vi "Duplicate_DO_WF.vi"(8 "error in":errorcluster) -> (0 "error out":errorcluster, 3 "Digital waveform 3":digitalwaveform[](graph))   [LabVIEW 2025]
uses:
  <vilib>/Waveform/DWDTOps.llb/DWDT Digital Size.vi
  <vilib>/Waveform/DWDTOps.llb/DWDT Append Digital Samples.vi
panel:
  out "Samples":u32
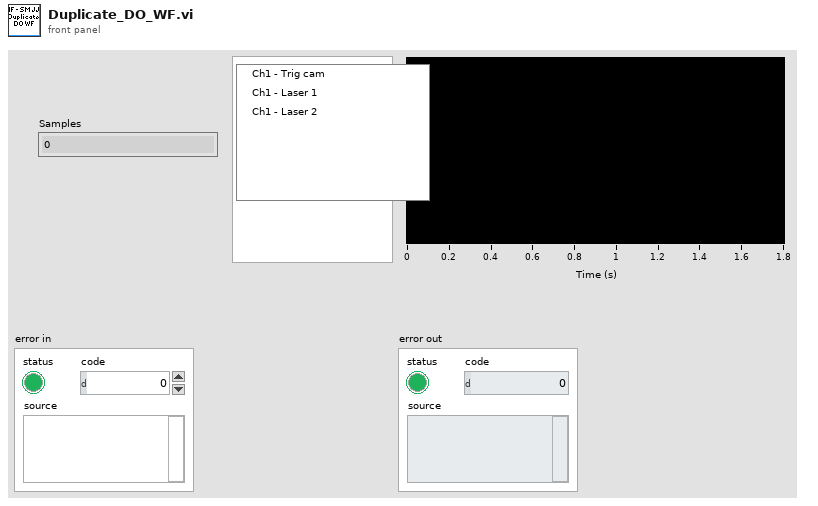
[diagram p1: front panel]
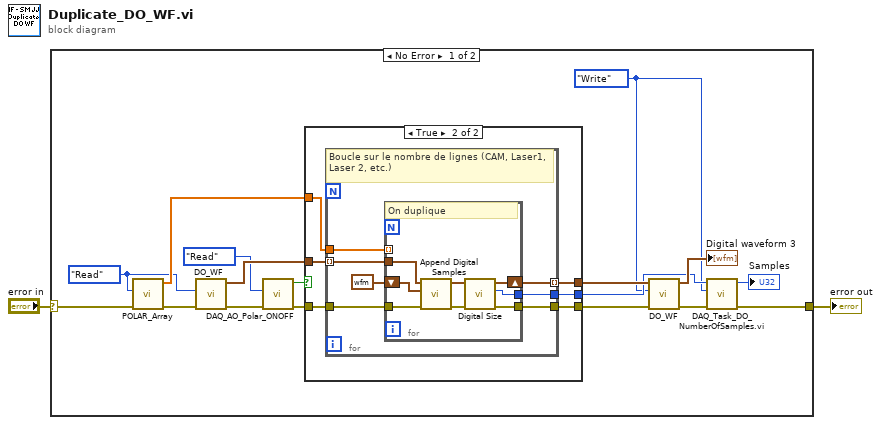
[diagram p0: block diagram]
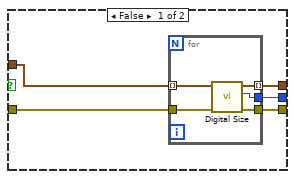
[diagram p2: hidden frame]
diagram:
  n1 = case shown="No Error" "error in" {
    selector: "error in" -> [w16 w51]
    tunnel: [w9 w51] -> w1
    frame No Error {
      w8 = enum16{"Init", "Write", "Read"}."Write" ("Action")
      w7 = enum16{"Init", "Write", "Read"}."Read" ("Action")
      n2 = call "POLAR_Array.vi"("error in"=w16, "Action"=w7) -> ("error out"=w15:errorcluster, "Pockels_Array"=w14:dbl[])  [unwired: 8 in]
      n3 = call "DO_WF.vi"("error in"=w15, "Action"=w7) -> ("error out"=w6:errorcluster, "Digital WF"=w19:digitalwaveform[])  [unwired: 8 in]
      n4 = call "DAQ_AO_Polar_ONOFF.vi"("error in"=w6, "Action"=enum16{"Init", "Write", "Read"}."Read") -> ("error out"=w5:errorcluster, "ON / OFF"=w3:bool)  [unwired: 8 in]
      n5 = case shown="True" w3 {
        tunnel: w19 -> [w24 w35]
        tunnel: [w22 w34] -> w18
        tunnel: w14 -> [_ w33]
        tunnel: [w20 w32] -> w13
        tunnel: [w23 w31] -> w12
        tunnel: w5 -> [w21 w30]
        frame False {
          n6 = for {
            tunnel: w24 -> [w29] mode=indexing
            tunnel: [w28] -> w23
            tunnel: [w27] -> w22
            tunnel: w21 -> [w26]
            tunnel: [w25] -> w20 mode=indexing
            n7 = call-poly <vilib>:"Digital Size.vi"("error in (no error)"=w26, "digital waveform in"=w29) -> ("error out"=w27:errorcluster, "number of samples"=w28:i32, "digital waveform out"=w25:digitalwaveform)  [unwired: 6 in, 1 out]
          }
        }
        frame True {
          n8 = for {
            tunnel: w35 -> [w42] mode=indexing
            tunnel: [w37] -> w32 mode=indexing
            tunnel: w33 -> [w40]
            tunnel: [w36] -> w31
            tunnel: w30 -> [w39]
            tunnel: [w38] -> w34
            # "Boucle sur le nombre de lignes (CAM, Laser1, Laser 2, etc.)"
            n9 = for {
              tunnel: w42 -> [w50]
              shift-right: [w43] -> w37
              shift-left: digitalwaveform {"t0"=timestamp(0 s since 1904-01-01), "dt"=1e-05, "Y"={"transitions"=[], "data"=[]}} ("digital waveform out") -> [w48]
              tunnel: w40 -> [_] mode=indexing
              tunnel: [w46] -> w36
              tunnel: w39 -> [w47]
              tunnel: [w44] -> w38
              # "On duplique"
              n10 = call-poly <vilib>:"Append Digital Samples.vi"("error in (no error)"=w47, "digital waveform B"=w48, "digital waveform A"=w50) -> ("error out"=w45:errorcluster, "digital waveform out"=w49:digitalwaveform)  [unwired: 7 in]
              n11 = call-poly <vilib>:"Digital Size.vi"("error in (no error)"=w45, "digital waveform in"=w49) -> ("error out"=w44:errorcluster, "number of samples"=w46:i32, "digital waveform out"=w43:digitalwaveform)  [unwired: 6 in, 1 out]
            }
          }
        }
      }
      n12 = call "DO_WF.vi"("error in"=w18, "Action"=w8, "Digital WF"=w13) -> ("error out"=w11:errorcluster, "Digital WF"=→"Digital waveform 3":digitalwaveform[])  [unwired: 7 in]
      n13 = call "DAQ_Task_DO_NumberOfSamples.vi.vi"("error in"=w11, "Action"=w8, "Samples"=w12) -> ("error out"=w9:errorcluster, "Samples"=→"Samples":u32)  [unwired: 7 in]
    }
    frame Error {
    }
  }
  "error out" <- w1
